vi "BooleanMeasure.vi"(5 "EndTime":timestamp, 7 "StartTime":timestamp, 8 "error in":errorcluster, 11 "BooleanMeasure":refnum<class "BooleanMeasure.lvclass">) -> (0 "error out":errorcluster, 3 "Passed":bool)   [LabVIEW 2020]
uses:
  <vilib>/Averna/ProligentResultProcessor/ProligentResultProcessor.lvlibp/Measure/BooleanMeasure/BooleanMeasure.lvclass
  <vilib>/Averna/ProligentResultProcessor/ProligentResultProcessor.lvlibp/Measure/Measure/Measure.lvclass
  C:/Program Files (x86)/National Instruments/LabVIEW 2020/vi.lib/Averna/ProligentResultProcessor/ProligentResultProcessor.lvlibp/Measure/Measure/Measure.lvclass
  C:/Program Files (x86)/National Instruments/LabVIEW 2020/vi.lib/Averna/ProligentResultProcessor/ProligentResultProcessor.lvlibp/Measure/BooleanMeasure/BooleanMeasure.lvclass
  <vilib>/Averna/ProligentResultProcessor/ProligentResultProcessor.lvlibp/Measure/MeasureLimit/MeasureLimit.lvclass
  <vilib>/Averna/ProligentResultProcessor/ProligentResultProcessor.lvlibp/Measure/BooleanMeasureLimit/BooleanMeasureLimit.lvclass
  C:/Program Files (x86)/National Instruments/LabVIEW 2020/vi.lib/Averna/ProligentResultProcessor/ProligentResultProcessor.lvlibp/Measure/MeasureLimit/MeasureLimit.lvclass
  C:/Program Files (x86)/National Instruments/LabVIEW 2020/vi.lib/Averna/ProligentResultProcessor/ProligentResultProcessor.lvlibp/Measure/BooleanMeasureLimit/BooleanMeasureLimit.lvclass
  <vilib>/Averna/ProligentResultProcessor/ProligentResultProcessor.lvlibp/Model/CustomData/CustomData.lvclass
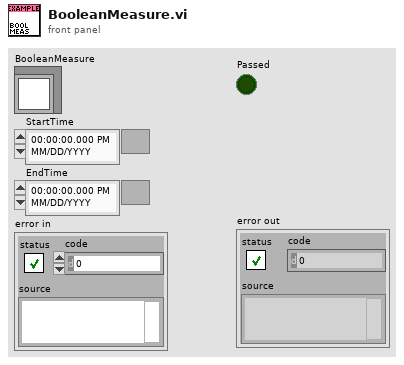
[diagram p1: front panel]
types:
  T1 = enum16{"PASS", "FAIL", "NOT_COMPLETED", "ABORTED"}
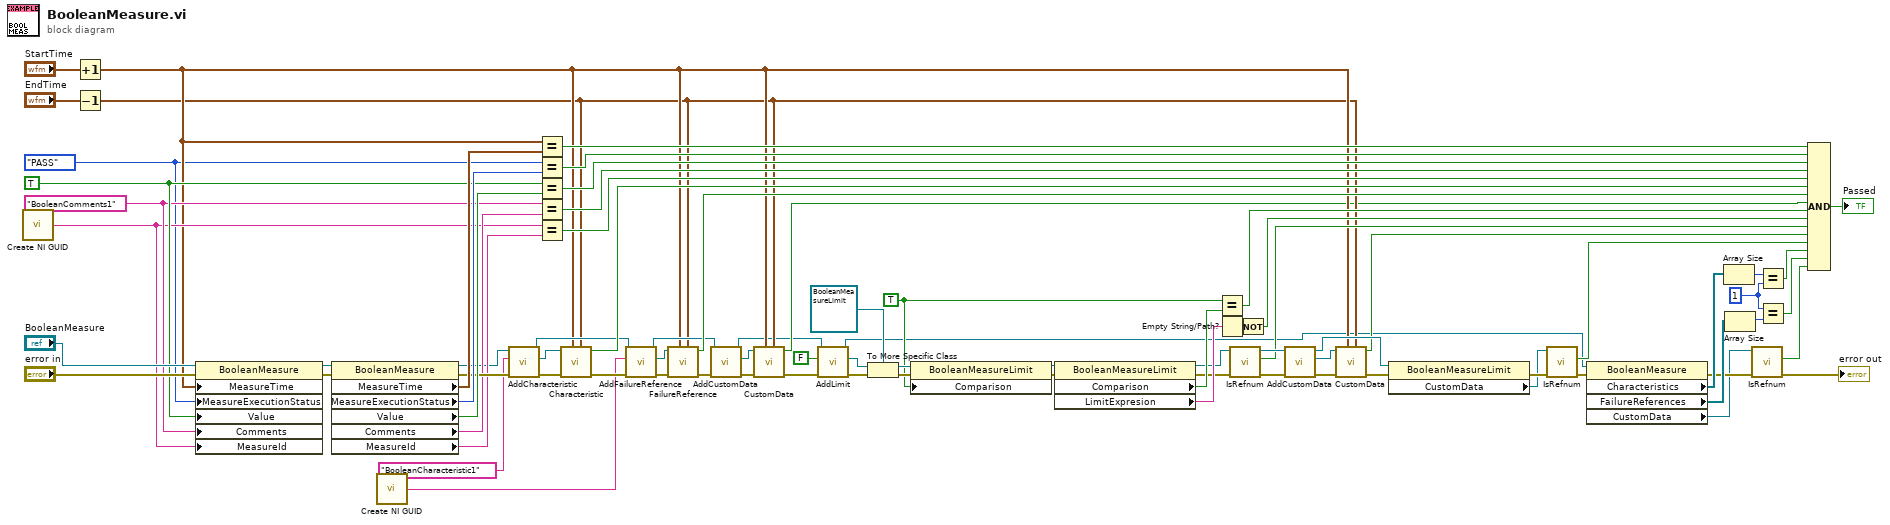
[diagram p0: block diagram]
diagram:
  w8 = 1 ("y")
  w42 = "BooleanComments1"
  w62 = TRUE ("Comparison")
  w70 = TRUE
  w17 = T1."PASS" ("ProcessRunStatus")
  n1 = call <vilib>:"Create NI GUID.vi"() -> ("NI GUID"=w40:string)
  n2 = Increment(x="StartTime") -> (x+1=w21:timestamp)
  n3 = Decrement(x="EndTime") -> (x-1=w20:timestamp)
  n4 = property class="BooleanMeasure"(reference="BooleanMeasure", error in="error in", "MeasureTime"=w21, "MeasureExecutionStatus"=w17, "Value"=w70, "Comments"=w42, "MeasureId"=w40) -> (reference out=w80:refnum<class "BooleanMeasure.lvclass">, error out=w79:errorcluster)
  n5 = property class="BooleanMeasure"(reference=w80, error in=w79) -> (reference out=w1:refnum<class "BooleanMeasure.lvclass">, error out=w69:errorcluster, "MeasureTime"=w78:timestamp, "MeasureExecutionStatus"=w77:T1, "Value"=w76:bool, "Comments"=w41:string, "MeasureId"=w39:string)
  n6 = call <vilib>:"Create NI GUID.vi"() -> ("NI GUID"=w28:string)
  n7 = call <vilib>:"AddCharacteristic.vi"("error in (no error)"=w69, "FullName"="BooleanCharacteristic1", "Measure in"=w1) -> ("error out"=w34:errorcluster, "Characteristic"=w32:refnum<class "Characteristic.lvclass">, "Measure out"=w29:refnum<class "BooleanMeasure.lvclass">)  [unwired: 6 in]
  n8 = Equal?(x=w21, y=w78) -> (x = y?=w75:bool)
  n9 = Equal?(x=w17, y=w77) -> (x = y?=w43:bool)
  n10 = Equal?(x=w70, y=w76) -> (x = y?=w74:bool)
  n11 = Equal?(x=w42, y=w41) -> (x = y?=w38:bool)
  n12 = Equal?(x=w40, y=w39) -> (x = y?=w37:bool)
  n13 = call "Characteristic.vi"("EndTime"=w20, "StartTime"=w21, "error in (no error)"=w34, "Characteristic in"=w32) -> ("error out"=w30:errorcluster, "Passed"=w31:bool)  [unwired: 6 in]
  n14 = call <vilib>:"AddFailureReference.vi"("error in (no error)"=w30, "Id"=w28, "Measure in"=w29) -> ("error out"=w16:errorcluster, "FailureReference"=w15:refnum<class "FailureReference.lvclass">, "Measure out"=w23:refnum<class "BooleanMeasure.lvclass">)  [unwired: 6 in]
  n15 = call "FailureReference.vi"("EndTime"=w20, "StartTime"=w21, "error in"=w16, "FailureReference"=w15) -> ("error out"=w27:errorcluster, "Passed"=w26:bool)  [unwired: 6 in]
  n16 = call <vilib>:"AddCustomData.vi"("error in (no error)"=w27, "Measure in"=w23) -> ("error out"=w24:errorcluster, "CustomData"=w22:refnum<class "CustomData.lvclass">, "Measure out"=w18:refnum<class "BooleanMeasure.lvclass">)  [unwired: 7 in]
  n17 = call "CustomData.vi"("EndTime"=w20, "StartTime"=w21, "error in"=w24, "CustomData"=w22) -> ("error out"=w25:errorcluster, "Passed"=w19:bool)  [unwired: 6 in]
  n18 = call <vilib>:"AddLimit.vi"("error in"=w25, "Comparison"=FALSE, "BooleanMeasure in"=w18) -> ("error out"=w35:errorcluster, "BooleanMeasureLimit"=w36:refnum<class "BooleanMeasureLimit.lvclass">, "BooleanMeasure out"=w13:refnum<class "BooleanMeasure.lvclass">)  [unwired: 6 in]
  n19 = To More Specific Class(target class=refnum<class "BooleanMeasureLimit.lvclass"> refnum ("ProligentResultProcessor:BooleanMeasureLimit"), reference=w36, error in=w35) -> (specific class reference=w65:refnum<class "BooleanMeasureLimit.lvclass">, error out=w67:errorcluster)
  n20 = property class="BooleanMeasureLimit"(reference=w65, error in=w67, "Comparison"=w62) -> (reference out=w64:refnum<class "BooleanMeasureLimit.lvclass">, error out=w63:errorcluster)
  n21 = property class="BooleanMeasureLimit"(reference=w64, error in=w63) -> (reference out=w52:refnum<class "BooleanMeasureLimit.lvclass">, error out=w57:errorcluster, "Comparison"=w61:bool, "LimitExpresion"=w60:string)
  n22 = Equal?(x=w62, y=w61) -> (x = y?=w59:bool)
  n23 = Empty String/Path?(string/path=w60) -> (empty?=w58:bool)
  n24 = call <vilib>:"IsRefnum.vi"("error in"=w57, "MeasureLimit in"=w52) -> ("error out"=w53:errorcluster, "IsRefnum"=w50:bool, "MeasureLimit out"=w51:refnum<class "BooleanMeasureLimit.lvclass">)  [unwired: 7 in]
  n25 = Not(x=w58) -> (.not. x?=w44:bool)
  n26 = call <vilib>:"AddCustomData.vi"("error in"=w53, "MeasureLimit in"=w51) -> ("error out"=w48:errorcluster, "CustomData"=w46:refnum<class "CustomData.lvclass">, "MeasureLimit out"=w49:refnum<class "BooleanMeasureLimit.lvclass">)  [unwired: 7 in]
  n27 = call "CustomData.vi"("EndTime"=w20, "StartTime"=w21, "error in"=w48, "CustomData"=w46) -> ("error out"=w47:errorcluster, "Passed"=w45:bool)  [unwired: 6 in]
  n28 = property class="BooleanMeasureLimit"(reference=w49, error in=w47) -> (error out=w56:errorcluster, "CustomData"=w55:refnum<class "CustomData.lvclass">)  [unwired: 1 out]
  n29 = call <vilib>:"IsRefnum.vi"("error in"=w56, "CustomDataType in"=w55) -> ("error out"=w14:errorcluster, "IsRefnum"=w54:bool)  [unwired: 7 in, 1 out]
  n30 = property class="BooleanMeasure"(reference=w13, error in=w14) -> (error out=w5:errorcluster, "Characteristics"=w12:refnum<class "Characteristic.lvclass">[], "FailureReferences"=w10:refnum<class "FailureReference.lvclass">[], "CustomData"=w3:refnum<class "CustomData.lvclass">)  [unwired: 1 out]
  n31 = Array Size(array=w12) -> (size(s)=w11:i32)
  n32 = Array Size(array=w10) -> (size(s)=w9:i32)
  n33 = call <vilib>:"IsRefnum.vi"("error in"=w5, "CustomDataType in"=w3) -> ("error out"=→"error out":errorcluster, "IsRefnum"=w2:bool)  [unwired: 7 in, 1 out]
  n34 = Equal?(x=w11, y=w8) -> (x = y?=w7:bool)
  n35 = Equal?(x=w8, y=w9) -> (x = y?=w6:bool)
  n36 = Compound Arithmetic op=AND(w75, w43, w74, w38, w37, w31, w26, w19, w59, w44, w50, w45, w54, w7, w6, w2) -> (→"Passed":bool)
